vi "TCPPacket Encode.vi"(8 "error in (no error)":errorcluster, 11 "TCPPacket in":refnum<class "TCPPacket.lvclass">) -> (0 "error out":errorcluster, 2 "Data":u8[](array[numeric]), 3 "TCPPacket out":refnum<class "TCPPacket.lvclass">)   [LabVIEW 2019, in "TCPPacket.lvclass"]
uses:
  TCPPacket.lvclass
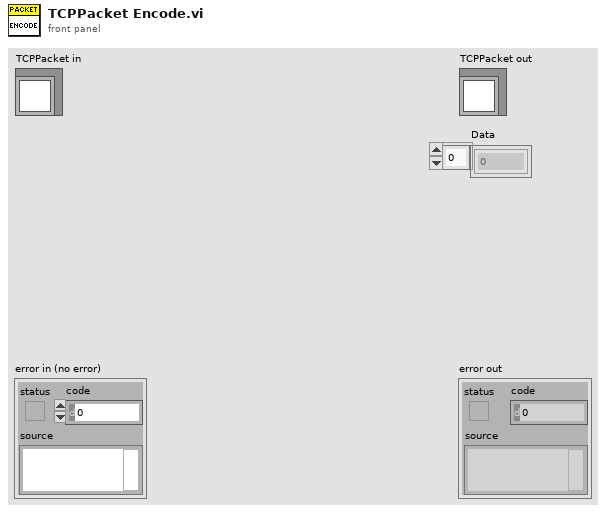
[diagram p1: front panel]
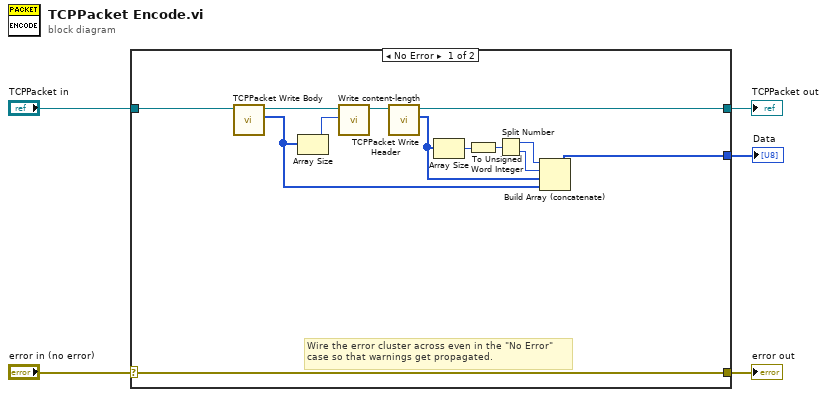
[diagram p0: block diagram]
diagram:
  n1 = case shown="No Error" "error in (no error)" {
    selector: "error in (no error)" -> [w18 w20]
    tunnel: [w18 w20] -> w4
    tunnel: [w16 w19] -> w2
    tunnel: "TCPPacket in" -> [w17 w19]
    tunnel: [w6 _] -> w1
    frame No Error {
      # "Wire the error cluster across even in the \"No Error\"\ncase so that warnings get propagated."
      n2 = call-dynamic "TCPPacket Write Body.vi"("TCPPacket in"=w17) -> ("Data"=w7:u8[], "TCPPacket out"=w15:refnum<class "TCPPacket.lvclass">)  [unwired: 8 in, 1 out]
      n3 = Array Size(array=w7) -> (size(s)=w13:i32)
      n4 = call-dynamic "Write content-length.vi"("content-length"=w13, "TCPPacket in"=w15) -> ("TCPPacket out"=w14:refnum<class "TCPPacket.lvclass">)  [unwired: 8 in, 1 out]
      n5 = call-dynamic "TCPPacket Write Header.vi"("TCPPacket in"=w14) -> ("Data"=w8:u8[], "TCPPacket out"=w16:refnum<class "TCPPacket.lvclass">)  [unwired: 8 in, 1 out]
      n6 = Array Size(array=w8) -> (size(s)=w12:i32)
      n7 = To Unsigned Word Integer(number=w12) -> (unsigned 16bit integer=w11:u16)
      n8 = Split Number(x=w11) -> (hi(x)=w9:u8, lo(x)=w10:u8)
      n9 = Build Array (concatenate)(w9, w10, w8, w7) -> (w6:u8[])
    }
    frame Error {
    }
  }
  "error out" <- w4
  "TCPPacket out" <- w2
  "Data" <- w1
